vi "Report Class Launch Result.vi"(1 "Object":refnum<class>, 3 "error in (no error)":errorcluster, 4 "Mode (Launch)":enum16{"Launch", "Terminate"}(ring)) -> (10 "error out":errorcluster)   [LabVIEW 2017]
doc: "Developed by Kevin Thompson\nkevin@thompsonengineering.net\n\nCopyright 2018-2020\nThompson Engineering, LLC"
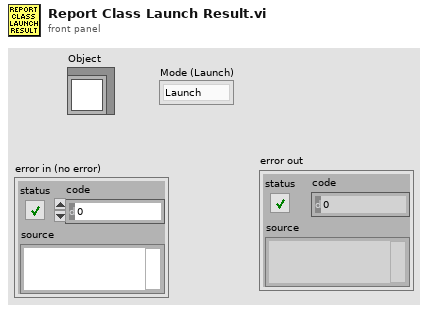
[diagram p1: front panel]
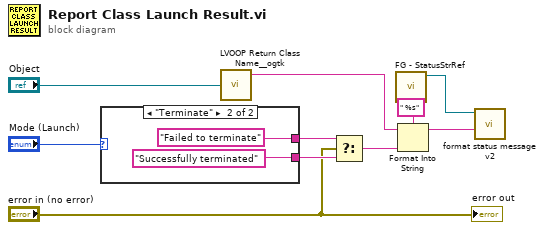
[diagram p0: block diagram]
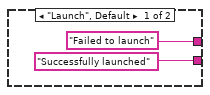
[diagram p2: hidden frame]
diagram:
  n1 = case shown="\"Terminate\"" "Mode (Launch)" {
    tunnel: ["Successfully launched" "Successfully terminated"] -> w5
    tunnel: ["Failed to launch" "Failed to terminate"] -> w4
    frame "Launch", Default {
    }
    frame "Terminate" {
    }
  }
  n2 = call <userlib>:"LVOOP Return Class Name__ogtk.vi"("Object"="Object") -> ("Class Base Name"=w9:string)  [unwired: 2 out]
  n3 = Select(t=w4, s="error in (no error)", f=w5) -> (s? t:f=w7:string)
  n4 = call "FG - StatusStrRef.vi"() -> ("StatusStr Ref out"=w10:refnum<vi>)  [unwired: 9 in, 1 out]
  n5 = Format Into String(format string=" %s", initial string=w9, w7) -> (resulting string=w8:string)  [unwired: 1 in, 1 out]
  n6 = call <vilib>:"format status message v2.vi"("status msg"=w8, "Str Refnum"=w10) -> ()  [unwired: 5 in, 5 out]
  "error out" <- "error in (no error)"
